vi "onGenerateStreamEvent.vi"(8 "error in (no error)":errorcluster, 9 "Direction":T1, 10 "Bytes":u8[](array[numeric]) format="%02x", 11 "DebuggingTerminal in":refnum<class "DebuggingTerminal.lvclass">) -> (0 "error out":errorcluster, 3 "DebuggingTerminal out":refnum<class "DebuggingTerminal.lvclass">)   [LabVIEW 2013, in "MQTT Base.lvlib" / "DebuggingTerminal.lvclass"]
uses:
  DebuggingTerminal.lvclass
  Stream Direction -- enum.ctl
  DebuggingTerminal.lvclass/DebuggingTerminal.ctl
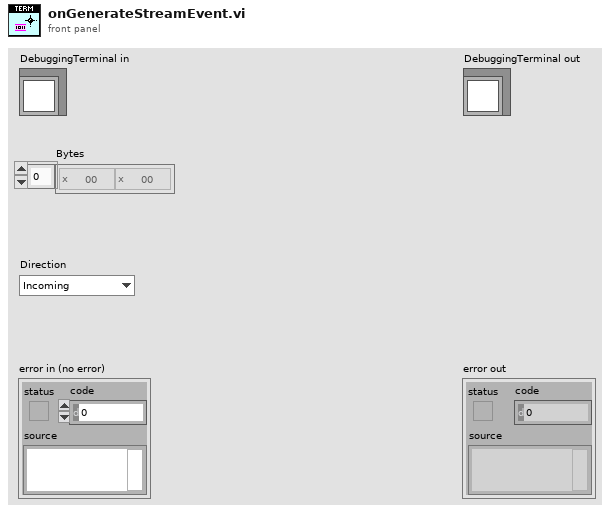
[diagram p1: front panel]
types:
  T1 = typedef "MQTT Base.lvlib/DebuggingTerminal.lvclass/Stream Direction -- enum.ctl" = enum16{"Incoming", "Outgoing"}
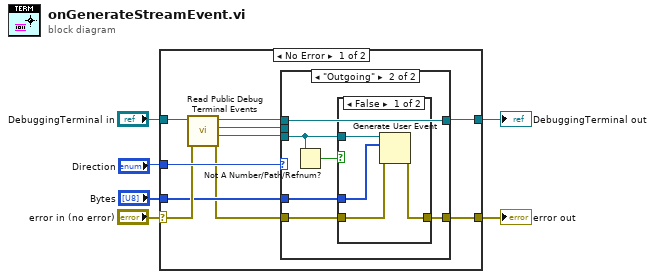
[diagram p0: block diagram]
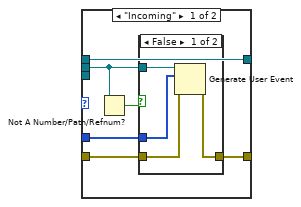
[diagram p2: hidden frame]
diagram:
  n1 = case shown="No Error" "error in (no error)" {
    selector: "error in (no error)" -> [w12 w40]
    tunnel: [w7 w40] -> w5
    tunnel: [w16 w39] -> w3
    tunnel: "DebuggingTerminal in" -> [w14 w39]
    tunnel: "Direction" -> [w15 _]
    tunnel: "Bytes" -> [w9 _]
    frame No Error {
      n2 = call "Read Public Debug Terminal Events.vi"("error in (no error)"=w12, "DebuggingTerminal in"=w14) -> ("error out"=w8:errorcluster, "Outgoing Stream"=w10:refnum<user-event>, "Incoming Stream"=w11:refnum<user-event>, "DebuggingTerminal out"=w13:refnum<class "DebuggingTerminal.lvclass">)  [unwired: 6 in]
      n3 = case shown="\"Outgoing\"" w15 {
        tunnel: [w22 w33] -> w16
        tunnel: w13 -> [w22 w33]
        tunnel: w11 -> [w21 _]
        tunnel: w10 -> [_ w29]
        tunnel: w9 -> [w19 w32]
        tunnel: w8 -> [w18 w31]
        tunnel: [w17 w30] -> w7
        frame "Incoming" {
          n4 = Not A Number/Path/Refnum?(number/path/refnum=w21) -> (NaN/Path/Refnum?=w20:bool)
          n5 = case shown="False" w20 {
            tunnel: w19 -> [w26 _]
            tunnel: w18 -> [w25 w27]
            tunnel: [w24 w27] -> w17
            tunnel: w21 -> [w23 _]
            frame False {
              n6 = Generate User Event(user event=w23, event data cluster=w26, error in=w25) -> (error out=w24:errorcluster)  [unwired: 1 in, 1 out]
            }
            frame True {
            }
          }
        }
        frame "Outgoing" {
          n7 = Not A Number/Path/Refnum?(number/path/refnum=w29) -> (NaN/Path/Refnum?=w28:bool)
          n8 = case shown="False" w28 {
            tunnel: w32 -> [w37 _]
            tunnel: w31 -> [w36 w38]
            tunnel: [w35 w38] -> w30
            tunnel: w29 -> [w34 _]
            frame False {
              n9 = Generate User Event(user event=w34, event data cluster=w37, error in=w36) -> (error out=w35:errorcluster)  [unwired: 1 in, 1 out]
            }
            frame True {
            }
          }
        }
      }
    }
    frame Error {
    }
  }
  "error out" <- w5
  "DebuggingTerminal out" <- w3
